vi "function generator host.vi"() -> ()   [LabVIEW 2009]
doc: "Use this template to measure or generate signals using the DAQ Assistant Express VI and NI-DAQmx. Double click the DAQ Assistant Express VI to launch a configuration wizard which steps you through configuring a measurement or generation.\n\nNote: You must have an NI-DAQmx compatible device installed to use this Express VI. Refer to the DAQ Quick Start Guide for NI-DAQ 7.0 for a list of compatible devices."
uses:
  <vilib>/rvi/interface/nirviOpenFPGA/nirviOpenFPGA.xnode
  FPGA Bitfiles/080509 FourPMT Det~96_FPGA Target 2_Streamlined FPGA--~5A.lvbitx
  FPGA Four PMTs/Streamlined FPGA--130415-3.vi
  <vilib>/FPGAPlugInAG/Pci-7833r/nirviIntfOpen_PCI-7833R.vi
  <vilib>/rvi/interface/nirviMethod/nirviMethod.xnode
  <vilib>/rvi/interface/common/niFpgaNodeNameForErrorReporting.ctl
  <vilib>/rvi/errors/niLvFpgaWhatHappensToTopLevelVI.ctl
  <vilib>/Utility/error.llb/Error Cluster From Error Code.vi
  <vilib>/rvi/errors/niLvFpgaAdjustHostInterfaceError.vi
  <vilib>/rvi/interface/nirviCloseFPGA/nirviCloseFPGA.xnode
  <vilib>/FPGAPlugInAG/Pci-7833r/nirviIntfClose_PCI-7833R.vi
  <vilib>/userDefined/High Color/nirio_resource_hc.ctl
  NiRioSrv.dll
panel:
  in  "stop":bool
  in  "Sorting amplitude [V]":dbl(knob)=1.0 min=0.0 max=10.0 step=0.1 scale=0.0..10.0
  in  "Output frequency [Hz]":u32(slide)=30000 min=1 step=1 scale=0.0..50000.0
  in  "Burst  cycles":i32(slide)=20 min=1 step=1 scale=0.0..1000.0
  in  "Sorting delay [us]":u32(slide)=100 step=100 scale=0.0..1000.0
  out "Sorting Pulse timetrace":cluster{dbl, dbl, dbl[]}(graph)
  # "Function Generator"
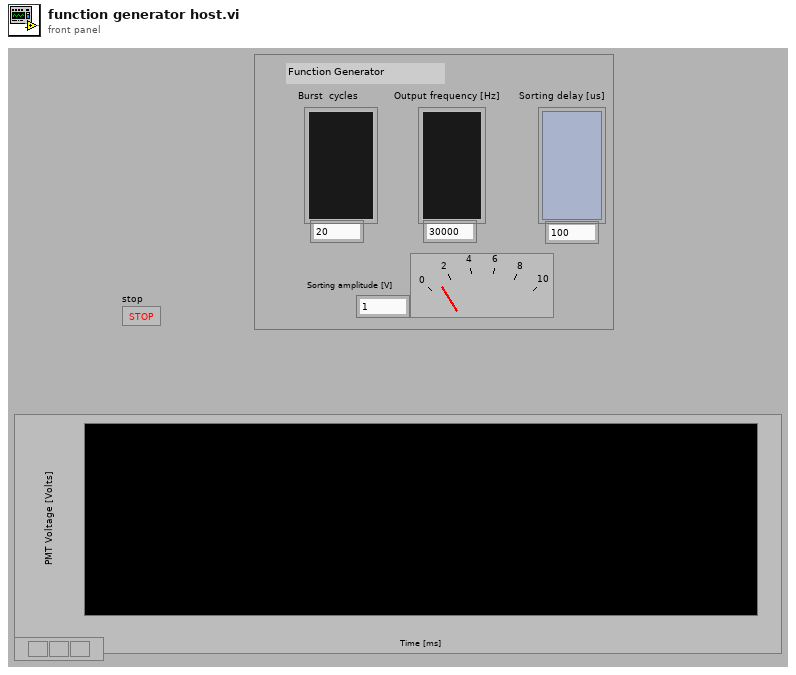
[diagram p1: front panel]
types:
  T1 = typedef "niFpgaNodeNameForErrorReporting.ctl" = enum16{"Open FPGA VI Reference", "Read/Write Control", "Invoke Method: Abort", "Invoke Method: Acknowledge IRQ", "Invoke Method: Download", "Invoke Method: FIFO.Configure", "Invoke Method: FIFO.Read", "Invoke Method: FIFO.Start", "Invoke Method: FIFO.Stop", "Invoke Method: FIFO.Write", "Invoke Method: Reset", "Invoke Method: Run", "Invoke Method: Wait on IRQ", "Close FPGA VI Reference"}
  T2 = typedef "niLvFpgaWhatHappensToTopLevelVI.ctl" = enum16{"top level VI scripted behind XNode", "top level VI inlined behind XNode"}
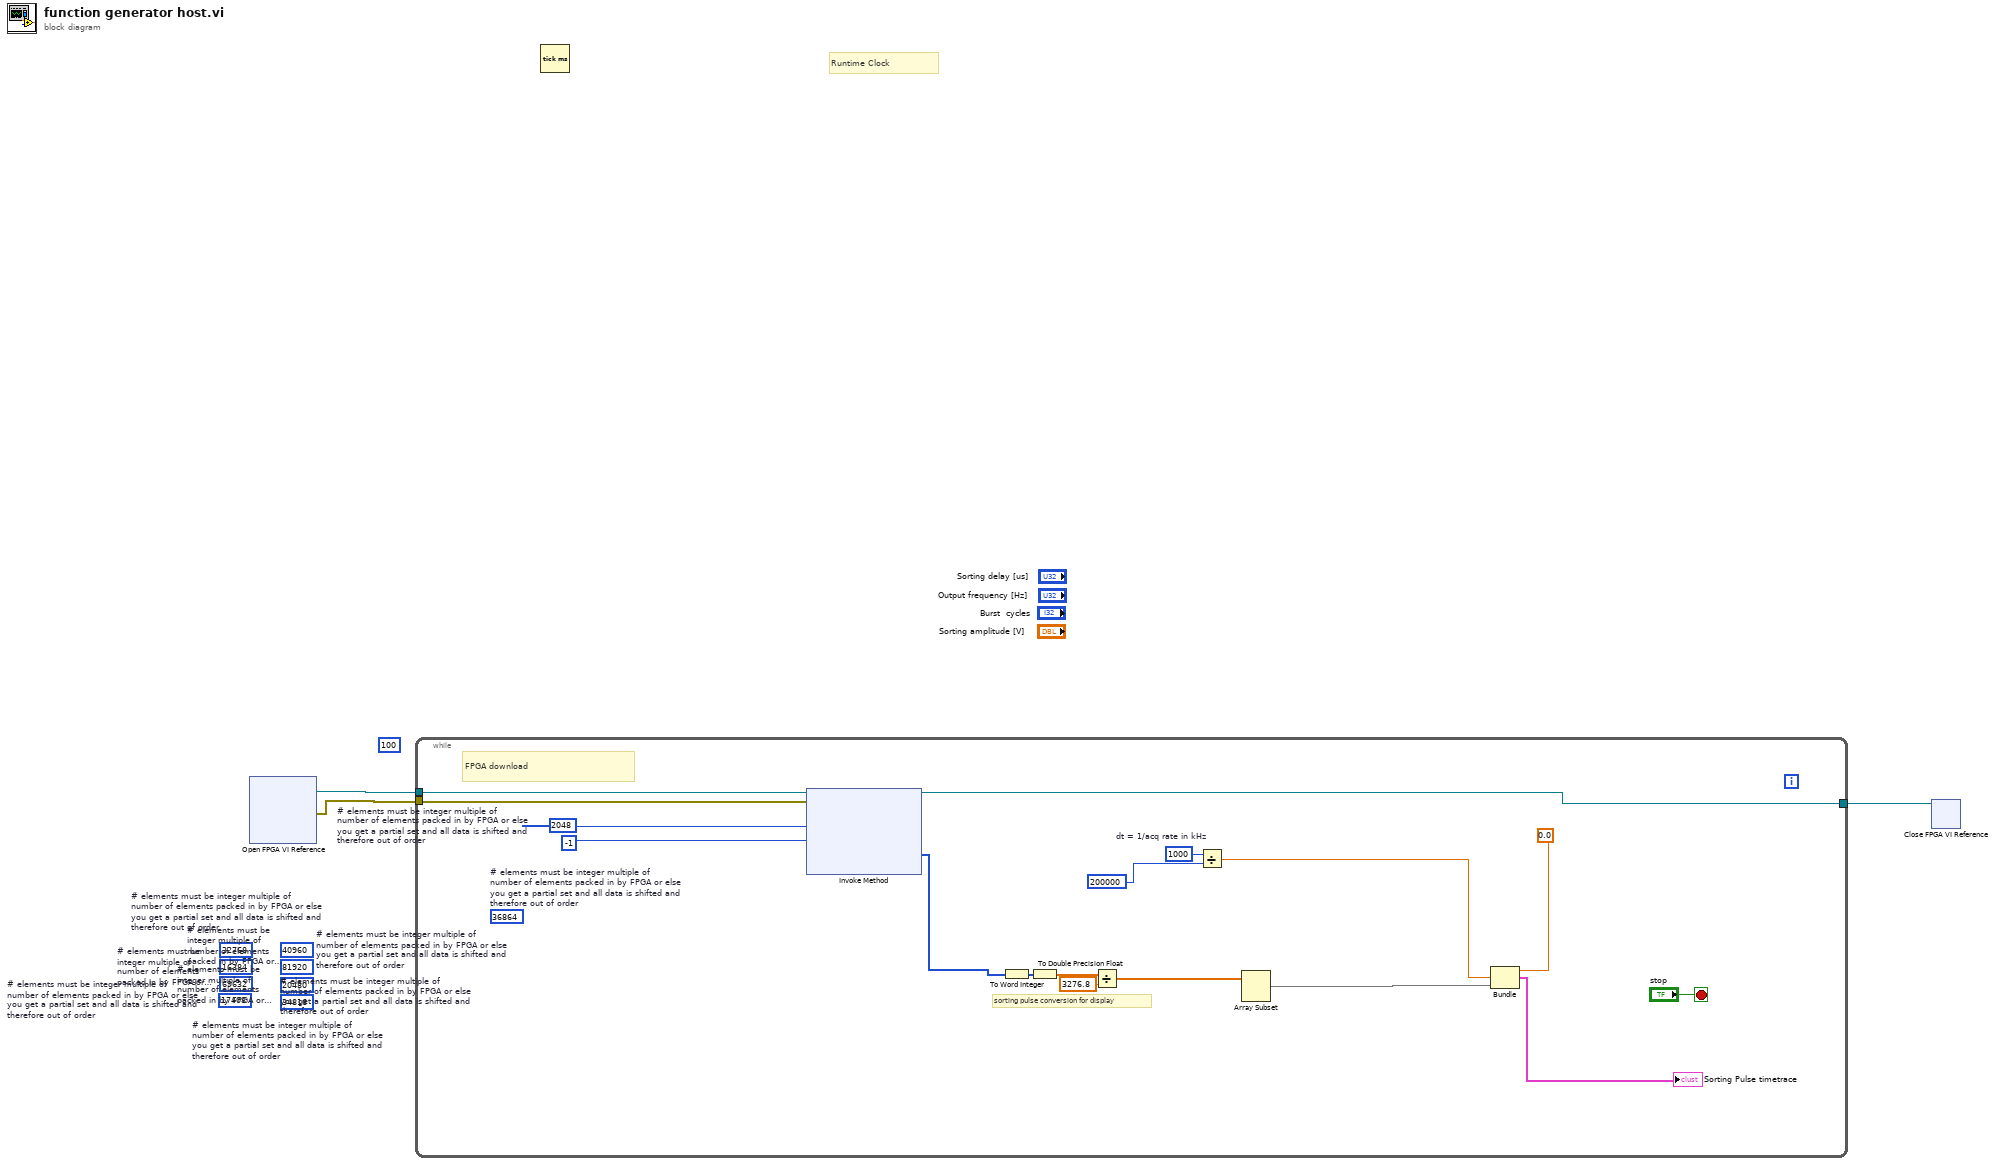
[diagram p0: block diagram]
diagram:
  (unwired) 100
  (unwired) u32 17408  # # elements must be integer multiple of number of elements packed in by FPGA or else you get a partial set and all data is shifted and therefore out of order
  (unwired) u32 69632  # # elements must be integer multiple of number of elements packed in by FPGA or else you get a partial set and all data is shifted and therefore out of order
  (unwired) u32 34816  # # elements must be integer multiple of number of elements packed in by FPGA or else you get a partial set and all data is shifted and therefore out of order
  (unwired) u32 40960  # # elements must be integer multiple of number of elements packed in by FPGA or else you get a partial set and all data is shifted and therefore out of order
  (unwired) u32 81920  # # elements must be integer multiple of number of elements packed in by FPGA or else you get a partial set and all data is shifted and therefore out of order
  (unwired) u32 20480  # # elements must be integer multiple of number of elements packed in by FPGA or else you get a partial set and all data is shifted and therefore out of order
  (unwired) u32 16384  # # elements must be integer multiple of number of elements packed in by FPGA or else you get a partial set and all data is shifted and therefore out of order
  (unwired) u32 32768  # # elements must be integer multiple of number of elements packed in by FPGA or else you get a partial set and all data is shifted and therefore out of order
  # "Runtime Clock"
  n1 = xnode "Open FPGA VI Reference"() -> ("FPGA VI Reference Out"=w3:refnum<k20>, "error out"=w2:errorcluster)  [unwired: 2 in]
  n2 = while {
    tunnel: w3 -> [w18]
    tunnel: w2 -> [w17]
    tunnel: [w4] -> w1
    stop <- "stop" stop-if-true
    (unwired) u32 36864  # # elements must be integer multiple of number of elements packed in by FPGA or else you get a partial set and all data is shifted and therefore out of order
    w20 = u32 2048  # # elements must be integer multiple of number of elements packed in by FPGA or else you get a partial set and all data is shifted and therefore out of order
    # "sorting pulse conversion for display"
    # "FPGA download"
    n3 = xnode "Invoke Method"("FPGA VI Reference In"=w18, "error in"=w17, "Number of Elements"=w20, "Timeout (ms)"=-1) -> ("FPGA VI Reference Out"=w4:refnum<k20>, "Data"=w6:i32[])  [unwired: 2 out]
    n4 = To Word Integer(number=w6) -> (16bit integer=w10:i16[])
    n5 = To Double Precision Float(number=w10) -> (double precision float=w9:dbl[])
    n6 = Divide(x=w9, y=3276.8) -> (x/y=w13:dbl[])
    n7 = Divide "dt = 1/acq rate in kHz"(x=1000, y=200000) -> (x/y=w8:dbl)
    n8 = Array Subset(array=w13) -> (w12:dbl[])  [unwired: 2 in]
    n9 = Bundle("x/y"=0.0, w8, w12) -> (→"Sorting Pulse timetrace":cluster{"x/y":dbl, dbl, dbl[]})  [unwired: 1 in]
  }
  n10 = Tick Count (ms)() -> ()  [unwired: 1 out]
  n11 = xnode "Close FPGA VI Reference"("FPGA VI Reference In"=w1) -> ()  [unwired: 1 in, 1 out]
